vi "GetDisplay.vi"(8 "error in (no error)":errorcluster, 11 "reference in":refnum<class "SceneRoot.lvclass">) -> (0 "error out":errorcluster, 2 "Display":refnum<vi>, 3 "reference out":refnum<class "SceneRoot.lvclass">)   [LabVIEW 2010, in "RenderBase.lvlib" / "SceneRoot.lvclass"]
uses:
  SceneRoot.lvclass
  SceneRoot.lvclass/SceneRoot.ctl
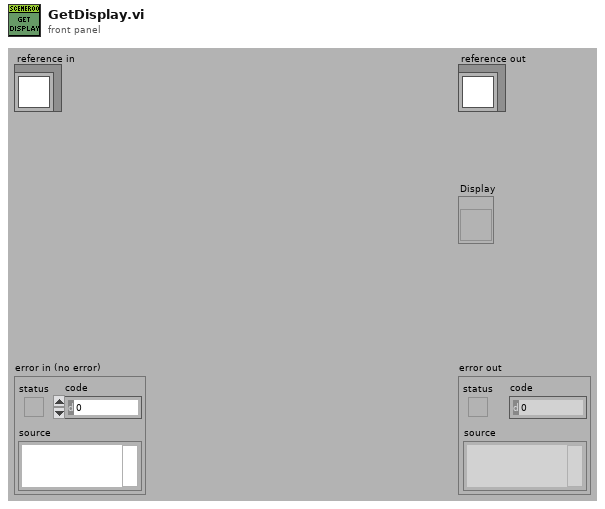
[diagram p1: front panel]
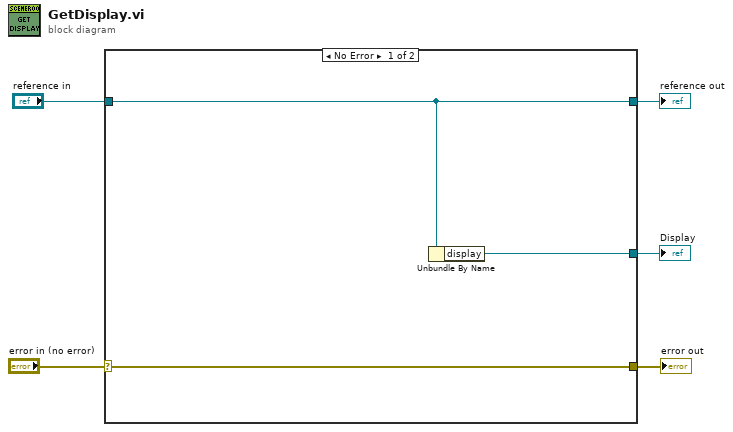
[diagram p0: block diagram]
diagram:
  n1 = case shown="No Error" "error in (no error)" {
    selector: "error in (no error)" -> [w6 w10]
    tunnel: [w6 w10] -> w4
    tunnel: [w8 w9] -> w2
    tunnel: "reference in" -> [w8 w9]
    tunnel: [w7 _] -> w1
    frame No Error {
      n2 = Unbundle By Name(w8) -> ("display"=w7:refnum<vi>)
    }
    frame Error {
    }
  }
  "error out" <- w4
  "reference out" <- w2
  "Display" <- w1
